vi "NewErrorCheck.vi"(11 "error in (no error)":errorcluster) -> (3 "Activate Script?":bool)   [LabVIEW 2024, in "Embedded TDMS Logger Engine.lvlib"]
uses:
  Embedded TDMS Logger Engine.lvlib
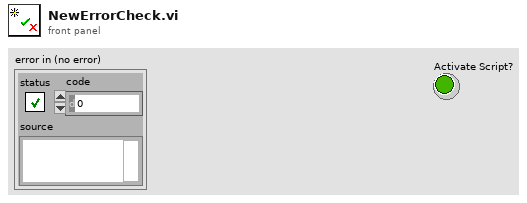
[diagram p1: front panel]
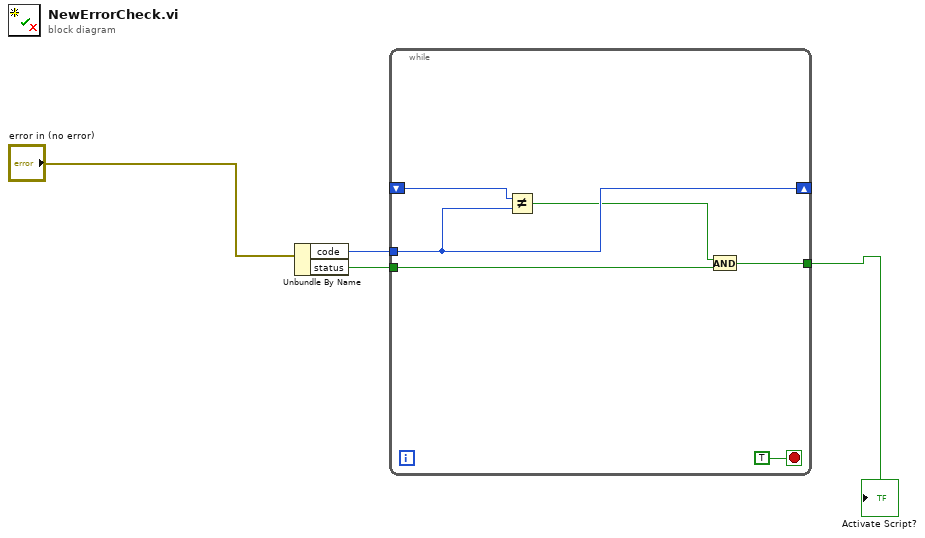
[diagram p0: block diagram]
diagram:
  n1 = Unbundle By Name("error in (no error)") -> ("code"=w1:i32, "status"=w3:bool)
  n2 = while {
    shift-right: [w6] -> _
    shift-left: _ -> [w7]
    tunnel: w3 -> [w9]
    tunnel: [w8] -> w2
    tunnel: w1 -> [w6]
    stop <- TRUE stop-if-true
    n3 = Not Equal?(x=w7, y=w6) -> (x != y?=w5:bool)
    n4 = And(x=w5, y=w9) -> (x .and. y?=w8:bool)
  }
  "Activate Script?" <- w2
